vi "calibratedIOField_facade.vi"(0 "Data In":T4, 2 "Display State In":T2={"calibration"=0.0, "unit"="m"}, 3 "Container State":T3) -> (6 "Data Out":T4, 7 "Display State Out":T2={"calibration"=0.0, "unit"="m"}, 8 "Action":T1)   [LabVIEW 2016, in "calibratedIOField.xctl"]
uses:
  calibratedIOField.xctl
  calibratedIOField_Data.ctl
  <vilib>/_xctls/Container State.ctl
  calibratedIOField_state.ctl
  <vilib>/_xctls/Action.ctl
  <vilib>/_xctls/XControlSupport.lvlib
panel:
  out "fieldIndicator":string
  in  "fieldControl":string
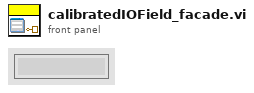
[diagram p1: front panel]
types:
  T1 = typedef "XControlSupport.lvlib/Action.ctl" = cluster{"Data Changed?":bool, "State Changed?":bool, "Action Name":string}
  T2 = typedef "calibratedIOField.xctl/calibratedIOField_state.ctl" = cluster{"calibration":dbl, "unit":string}
  T3 = typedef "XControlSupport.lvlib/Container State.ctl" = cluster{"Indicator?":bool, "Run Mode?":bool, " Refnum":refnum<vi>}
  T4 = typedef "calibratedIOField.xctl/calibratedIOField_Data.ctl" = dbl
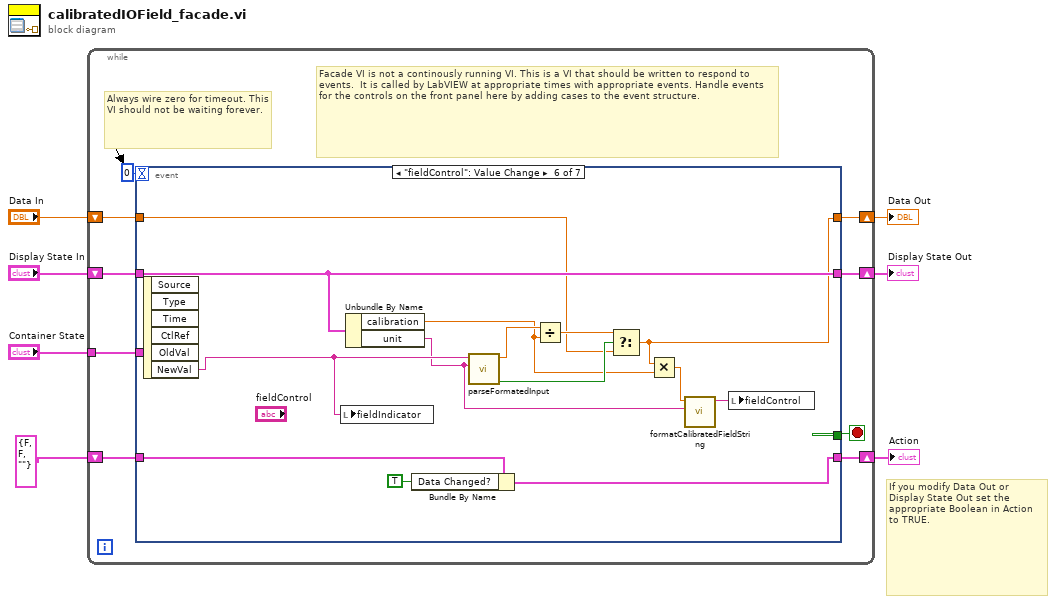
[diagram p0: block diagram]
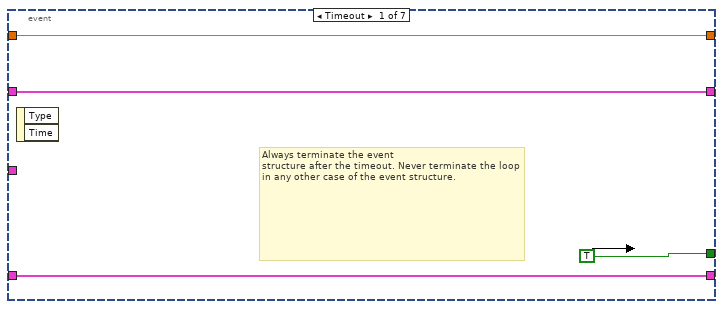
[diagram p2: hidden frame]
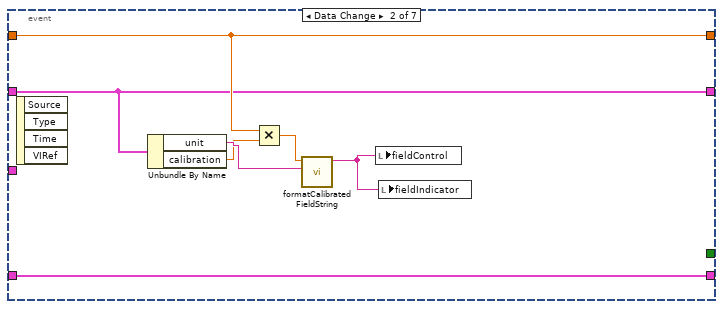
[diagram p3: hidden frame]
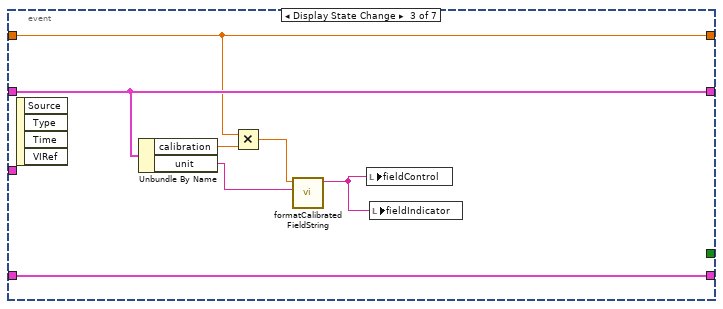
[diagram p4: hidden frame]
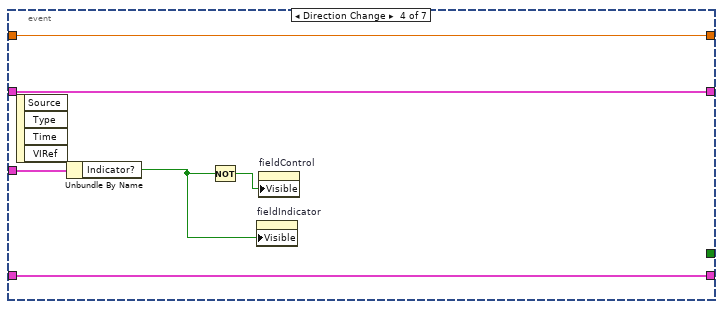
[diagram p5: hidden frame]
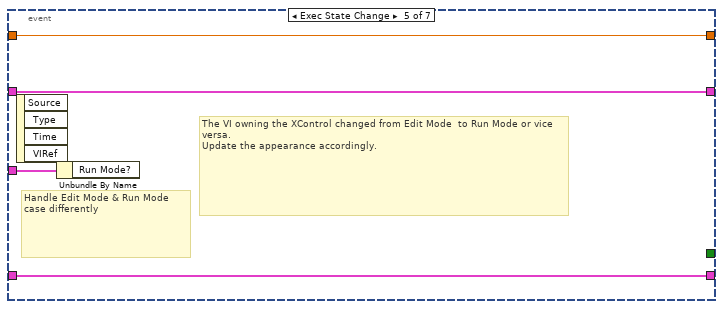
[diagram p6: hidden frame]
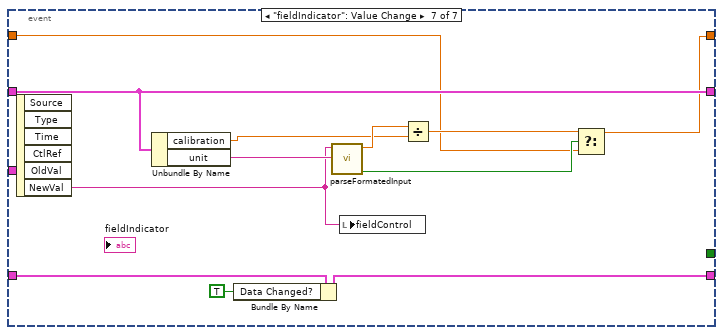
[diagram p7: hidden frame]
diagram:
  # "If you modify Data Out or\nDisplay State Out set the\nappropriate Boolean in Action\nto TRUE."
  n1 = while {
    shift-right: [w15] -> w4
    shift-left: "Display State In" -> [w16]
    tunnel: "Container State" -> [w12]
    shift-right: [w10] -> w7
    shift-left: "Data In" -> [w11]
    shift-right: [w8] -> w2
    shift-left: T1 {"Data Changed?"=FALSE, "State Changed?"=FALSE, "Action Name"=""} ("Action") -> [w9]
    stop <- w14 stop-if-true
    # "Facade VI is not a continously running VI. This is a VI that should be written to respond to events.  It is called by LabVIEW at appropriate times with appropriate events. Handle events for the controls on the front panel here by adding cases to the event structure."
    # "Always wire zero for timeout. This\nVI should not be waiting forever."
    n2 = event shown="[5] \"fieldControl\": Value Change" {
      selector: _ -> [_ _ _ _ _ _ _]
      dyn-events: _ -> [_ _ _ _ _ _ _]
      timeout: 0 -> [_ _ _ _ _ _ _]
      tunnel: w16 -> [w18 w25 w31 w39 w43 w58 w69]
      tunnel: [w18 w25 w31 w39 w43 w58 w69] -> w15
      tunnel: [TRUE _ _ _ _ _ _] -> w14
      tunnel: w12 -> [_ _ _ w40 w44 _ _]
      tunnel: w11 -> [w17 w26 w30 w38 w42 w54 w62]
      tunnel: [w17 w26 w30 w38 w42 w51 w64] -> w10
      tunnel: [w19 w27 w34 w37 w41 w48 w60] -> w8
      tunnel: w9 -> [w19 w27 w34 w37 w41 w49 w70]
      event Timeout {
        # "Always terminate the event\nstructure after the timeout. Never terminate the loop in any other case of the event structure."
        n3 = event-data() -> ()  [unwired: 1 in, 2 out]
      }
      event Data Change {
        n4 = event-data() -> ()  [unwired: 1 in, 4 out]
        n5 = Unbundle By Name(w25) -> ("unit"=w24:string, "calibration"=w21:dbl)
        n6 = Multiply(x=w26, y=w21) -> (x*y=w22:T4)
        n7 = call "formatCalibratedFieldString.vi"("unit"=w24, "numIn"=w22) -> ("formatedNumber"=w23:string)  [unwired: 9 in]
        n8 = local write "fieldControl"(w23) -> ()
        n9 = local write "fieldIndicator"(w23) -> ()
      }
      event Display State Change {
        n10 = event-data() -> ()  [unwired: 1 in, 4 out]
        n11 = Unbundle By Name(w31) -> ("calibration"=w28:dbl, "unit"=w33:string)
        n12 = Multiply(x=w30, y=w28) -> (x*y=w29:T4)
        n13 = call "formatCalibratedFieldString.vi"("unit"=w33, "numIn"=w29) -> ("formatedNumber"=w32:string)  [unwired: 9 in]
        n14 = local write "fieldControl"(w32) -> ()
        n15 = local write "fieldIndicator"(w32) -> ()
      }
      event Direction Change {
        n16 = event-data() -> ()  [unwired: 1 in, 4 out]
        n17 = Unbundle By Name(w40) -> ("Indicator?"=w36:bool)
        n18 = Not(x=w36) -> (.not. x?=w35:bool)
        n19 = property on="fieldIndicator" class="Str"("Visible"=w36) -> ()  [unwired: 2 in, 2 out]
        n20 = property on="fieldControl" class="Str"("Visible"=w35) -> ()  [unwired: 2 in, 2 out]
      }
      event Exec State Change {
        # "The VI owning the XControl changed from Edit Mode  to Run Mode or vice versa.\nUpdate the appearance accordingly."
        # "Handle Edit Mode & Run Mode\ncase differently"
        n21 = event-data() -> ()  [unwired: 1 in, 4 out]
        n22 = Unbundle By Name(w44) -> ()  [unwired: 1 out]
      }
      event "fieldControl": Value Change {
        n23 = event-data() -> ("NewVal"=w53:string)  [unwired: 1 in, 5 out]
        n24 = local write "fieldIndicator"(w53) -> ()
        n25 = Unbundle By Name(w58) -> ("calibration"=w45:dbl, "unit"=w52:string)
        n26 = Bundle By Name(cluster=w49, "Data Changed?"=TRUE) -> (w48:T1)
        n27 = call "parseFormatedInput.vi"("unit"=w52, "inputString"=w53) -> ("matchValid"=w55:bool, "parsedNumber"=w57:dbl)  [unwired: 8 in]
        n28 = Divide(x=w57, y=w45) -> (x/y=w56:dbl)
        n29 = Select(t=w56, s=w55, f=w54) -> (s? t:f=w51:T4)
        n30 = Multiply(x=w51, y=w45) -> (x*y=w46:T4)
        n31 = call "formatCalibratedFieldString.vi"("unit"=w52, "numIn"=w46) -> ("formatedNumber"=w50:string)  [unwired: 9 in]
        n32 = local write "fieldControl"(w50) -> ()
      }
      event "fieldIndicator": Value Change {
        n33 = event-data() -> ("NewVal"=w61:string)  [unwired: 1 in, 5 out]
        n34 = Unbundle By Name(w69) -> ("calibration"=w65:dbl, "unit"=w68:string)
        n35 = Bundle By Name(cluster=w70, "Data Changed?"=TRUE) -> (w60:T1)
        n36 = call "parseFormatedInput.vi"("unit"=w68, "inputString"=w61) -> ("matchValid"=w63:bool, "parsedNumber"=w66:dbl)  [unwired: 8 in]
        n37 = local write "fieldControl"(w61) -> ()
        n38 = Divide(x=w66, y=w65) -> (x/y=w67:dbl)
        n39 = Select(t=w67, s=w63, f=w62) -> (s? t:f=w64:T4)
      }
    }
  }
  "Display State Out" <- w4
  "Data Out" <- w7
  "Action" <- w2
